vi "19.2.2-QR Code.vi"() -> ()   [LabVIEW 2017]
doc: "This example illustrates how to use the Read QR Code VI. There are several types of QR codes that are supported including Micro, Model 1 and Model 2, as well as various cell shapes and barcode shapes."
uses:
  <vilib>/vision/Instrument.llb/QR Code Description Options.ctl
  <vilib>/vision/Instrument.llb/Data Matrix Polarity.ctl
  <vilib>/vision/Instrument.llb/QR Code Model Type.ctl
  <vilib>/vision/Instrument.llb/QR Code Search Options.ctl
  <vilib>/vision/Instrument.llb/Demodulation Mode.ctl
  <vilib>/vision/Instrument.llb/Cell Sample Size.ctl
  <vilib>/vision/Instrument.llb/Cell Filter Mode.ctl
  <vilib>/vision/NI_Vision_Development_Module.lvlib
panel:
  out "Read Time (ms)":dbl format="%.2f"
  out "Data:":string
  out "Image":T1(plugin-control)
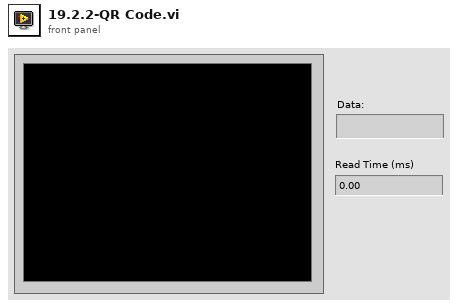
[diagram p1: front panel]
types:
  T1 = typedef "IMAQ Image.ctl" = refnum<image>
  T2 = typedef "Image Type" = u32
  T3 = typedef "QR Code Search Options.ctl" = cluster{"Rotation Mode":enum32{"Unlimited", "0 Degrees", "90 Degrees", "180 Degrees", "270 Degrees"}, "Skip Location?":bool, "Edge Threshold":u32, "Demodulation Mode":T4, "Cell Sample Size":T5, "Cell Filter Mode":T6, "Skew Degrees Allowed":u32}
  T4 = typedef "Demodulation Mode.ctl" = i32
  T5 = typedef "Cell Sample Size.ctl" = i32
  T6 = typedef "Cell Filter Mode.ctl" = i32
  T7 = typedef "QR Code Description Options.ctl" = cluster{"Matrix Size (cells)":i32, "Barcode Polarity":T8, "Mirror Mode":i32, "QR Model":T9}
  T8 = typedef "Data Matrix Polarity.ctl" = i32
  T9 = typedef "QR Code Model Type.ctl" = i32
  T10 = typedef "QR Code Report.ctl" = cluster{"Found?":bool, "Data":string, "Bounding Box":cluster{"x":sgl, "y":sgl}[], "Errors Corrected":u32, "Dimensions (Rows/Cols)":u32, "Version":u32, "QR Model":T9, "Stream Mode":T11, "Barcode Polarity":T8, "Mirrored?":bool, "Append Stream Position":u32, "Size of Append Stream":u32, "First EAN-128 ID":i32, "First Alternate Language ID":i32, "Append Stream ID":u32, "Minimum Edge Strength":u32, "Demodulation Mode":T4, "Cell Sample Size":T5, "Cell Filter Mode":T6}
  T11 = typedef "QR Code Stream Mode Type.ctl" = i32
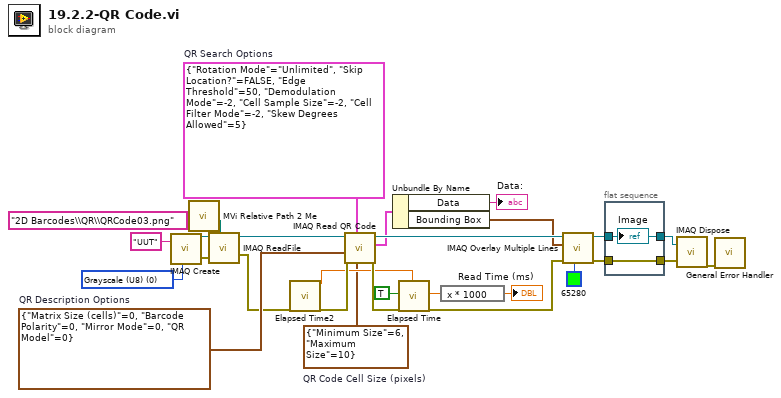
[diagram p0: block diagram]
diagram:
  w6 = T2 0 items=["Grayscale (U8)", "Grayscale (I16)", "Grayscale (SGL)", "Complex (CSG)", "RGB (U32)", "HSL (U32)", "RGB (U64)", "Grayscale (U16)"] ("Image Type")
  w17 = T3 {"Rotation Mode"=enum."Unlimited", "Skip Location?"=FALSE, "Edge Threshold"=50, "Demodulation Mode"=-2, "Cell Sample Size"=-2, "Cell Filter Mode"=-2, "Skew Degrees Allowed"=5}  # QR Search Options
  w16 = T7 {"Matrix Size (cells)"=0, "Barcode Polarity"=0, "Mirror Mode"=0, "QR Model"=0}  # QR Description Options
  w15 = cluster{"Minimum Size":u32, "Maximum Size":u32} {"Minimum Size"=6, "Maximum Size"=10}  # QR Code Cell Size (pixels)
  n1 = call "IMAQ Create"("Image Name"="UUT", "Image Type"=w6) -> ("New Image"=w8:T1, "error out"=w7:errorcluster)  [unwired: 3 in]
  n2 = call "MVi Relative Path 2 Me.vi"("Relative Path"="2D Barcodes\\QR\\QRCode03.png") -> ("Appended Dir"=w11:path)  [unwired: 5 in, 1 out]
  n3 = call "IMAQ ReadFile"("File Path"=w11, "error in (no error)"=w7, "Image"=w8) -> ("error out"=w9:errorcluster, "Image Out"=w10:T1)  [unwired: 4 in, 3 out]
  n4 = call "Elapsed Time2"("error in (no error)"=w9) -> ("Present (s)"=w19:dbl, "error out"=w22:errorcluster)  [unwired: 11 in, 6 out]
  n5 = call "IMAQ Read QR Code"("QR Code Cell Size (pixels)"=w15, "QR Search Options"=w17, "error in (no error)"=w22, "QR Description Options"=w16, "Image"=w10) -> ("error out"=w21:errorcluster, "QR Code Report"=w23:T10, "Image (duplicate)"=w24:T1)  [unwired: 3 in, 1 out]
  n6 = Unbundle By Name(w23) -> ("Data"=→"Data:":string, "Bounding Box"=w14:cluster{"x":sgl, "y":sgl}[])
  n7 = call "Elapsed Time"("Reset"=TRUE, "error in (no error)"=w21, "Set Start Time (s)"=w19) -> ("Elapsed Time (s)"=w26:dbl, "error out"=w20:errorcluster)  [unwired: 9 in, 6 out]
  n8 = expression code="x * 1000"(w26) -> (→"Read Time (ms)":dbl)
  n9 = call "IMAQ Overlay Multiple Lines"("Color"=u32 65280, "error in (no error)"=w20, "Line End Points"=w14, "Image"=w24) -> ("error out"=w2:errorcluster, "Image Out"=w28:T1)  [unwired: 6 in]
  n10 = flat-sequence {
    tunnel: w28 -> [w30]
    tunnel: [w30] -> w3
    tunnel: w2 -> [w29]
    tunnel: [w29] -> w1
    frame #0 {
      "Image" <- w30
    }
  }
  n11 = call "IMAQ Dispose"("Image"=w3, "error in (no error)"=w1) -> ("error out"=w4:errorcluster)  [unwired: 4 in]
  n12 = call <vilib>:"General Error Handler.vi"("error in (no error)"=w4) -> ()  [unwired: 10 in, 5 out]
